vi "Send_Message.vi"(0 "session in":refnum<k35>, 5 "board":u8 format="%x", 7 "Send Message":T1 {"Command" format="%x"; "dst" format="%x"}, 11 "error in (no error)":errorcluster) -> (4 "session out":refnum<k35>, 8 "Message":string, 15 "error out":errorcluster)   [LabVIEW 2021]
uses:
  Controles/Send_Message.ctl
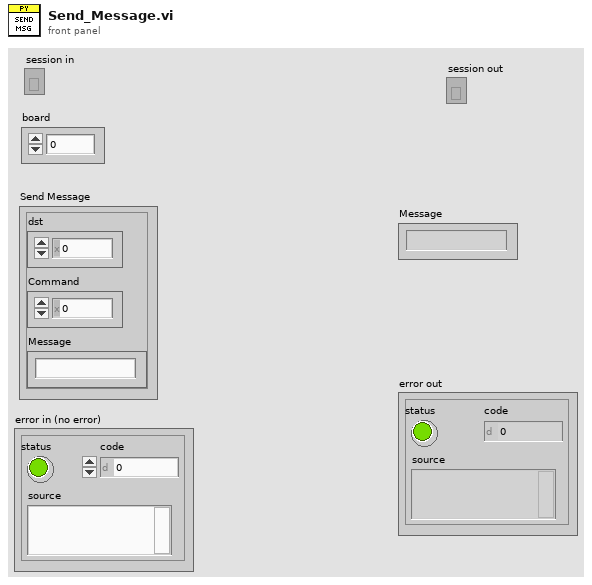
[diagram p1: front panel]
types:
  T1 = typedef "Send_Message.ctl" = cluster{"dst":i64, "Command":i64, "Message":string}
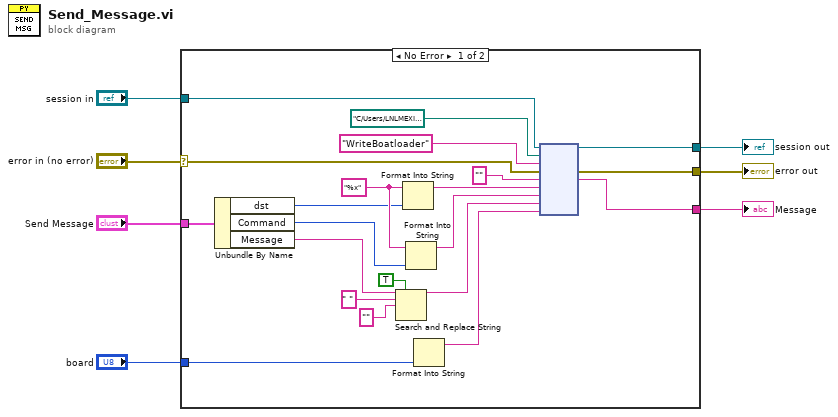
[diagram p0: block diagram]
diagram:
  n1 = case shown="No Error" "error in (no error)" {
    selector: "error in (no error)" -> [w15 w29]
    tunnel: "board" -> [w23 _]
    tunnel: "session in" -> [w22 w30]
    tunnel: [w21 w30] -> w5
    tunnel: [w20 w29] -> w4
    tunnel: "Send Message" -> [w12 _]
    tunnel: [w8 _] -> w1
    frame No Error {
      w14 = "%x" ("format string")
      n2 = Unbundle By Name(w12) -> ("dst"=w11:i64, "Command"=w10:i64, "Message"=w9:string)
      n3 = Search and Replace String(replace all?=TRUE ("replace all? (F)"), input string=w9, search string=" ", replace string="" ("replace string (\"\")")) -> (result string=w13:string)  [unwired: 4 in, 3 out]
      n4 = Format Into String(format string=w14, w11) -> (resulting string=w25:string)  [unwired: 2 in, 1 out]
      n5 = Format Into String(format string=w14, w10) -> (resulting string=w24:string)  [unwired: 2 in, 1 out]
      n6 = Format Into String(w23) -> (resulting string=w19:string)  [unwired: 3 in, 1 out]
      n7 = node(w22, path "C:/Users/LNLMEXID/Desktop/GEA3 Python/Main.py" ("module path"), "WriteBoatloader" ("function name"), w15, "" ("data_hex"), w25, w24, w13, w19) -> (w21:refnum<k35>, w20:errorcluster, w8:string)  [unwired: 4 in, 2 out]
    }
    frame Error {
    }
  }
  "session out" <- w5
  "error out" <- w4
  "Message" <- w1
